vi "Send8Bytes.vi"(0 "data0":u8, 1 "data1":u8, 2 "data2":u8, 3 "data3":u8, 4 "data4":u8, 5 "data5":u8, 6 "data6":u8, 7 "data7":u8, 8 "类型":u32(ring)=4 items=["PCI5121"=1, "PCI9810"=2, "USBCAN1"=3, "USBCAN2"=4, "PCI9820"=5, "CAN232"=6, "PCI5110"=7, "CANLite(mini)"=8, "ISA9620"=9, "ISA5420"=10, "PC104CAN"=11, "CANET"=17, "DNP9810"=13, "USBCAN-E-U"=20, "USBCAN-2E-U"=21], 9 "板号/目标地址":u8, 10 "设备索引":u32(ring) items=["0", "1", "2", "3", "4", "5", "6", "7", "8", "9", "10", "11", "12", "13", "14", "15", ""], 12 "CAN路数":u32(ring) items=["0", "1"], 14 "ExternFlag":u8, 16 "ID":u32, 18 "DataLen":u8) -> (20 "发送状态":bool)   [LabVIEW 2013]
uses:
  BHN01/AutoBurn/Settings/ControlCAN.dll
panel:
  out "VCI_CAN_OBJ_T":T1 {"ID" format="%x"}
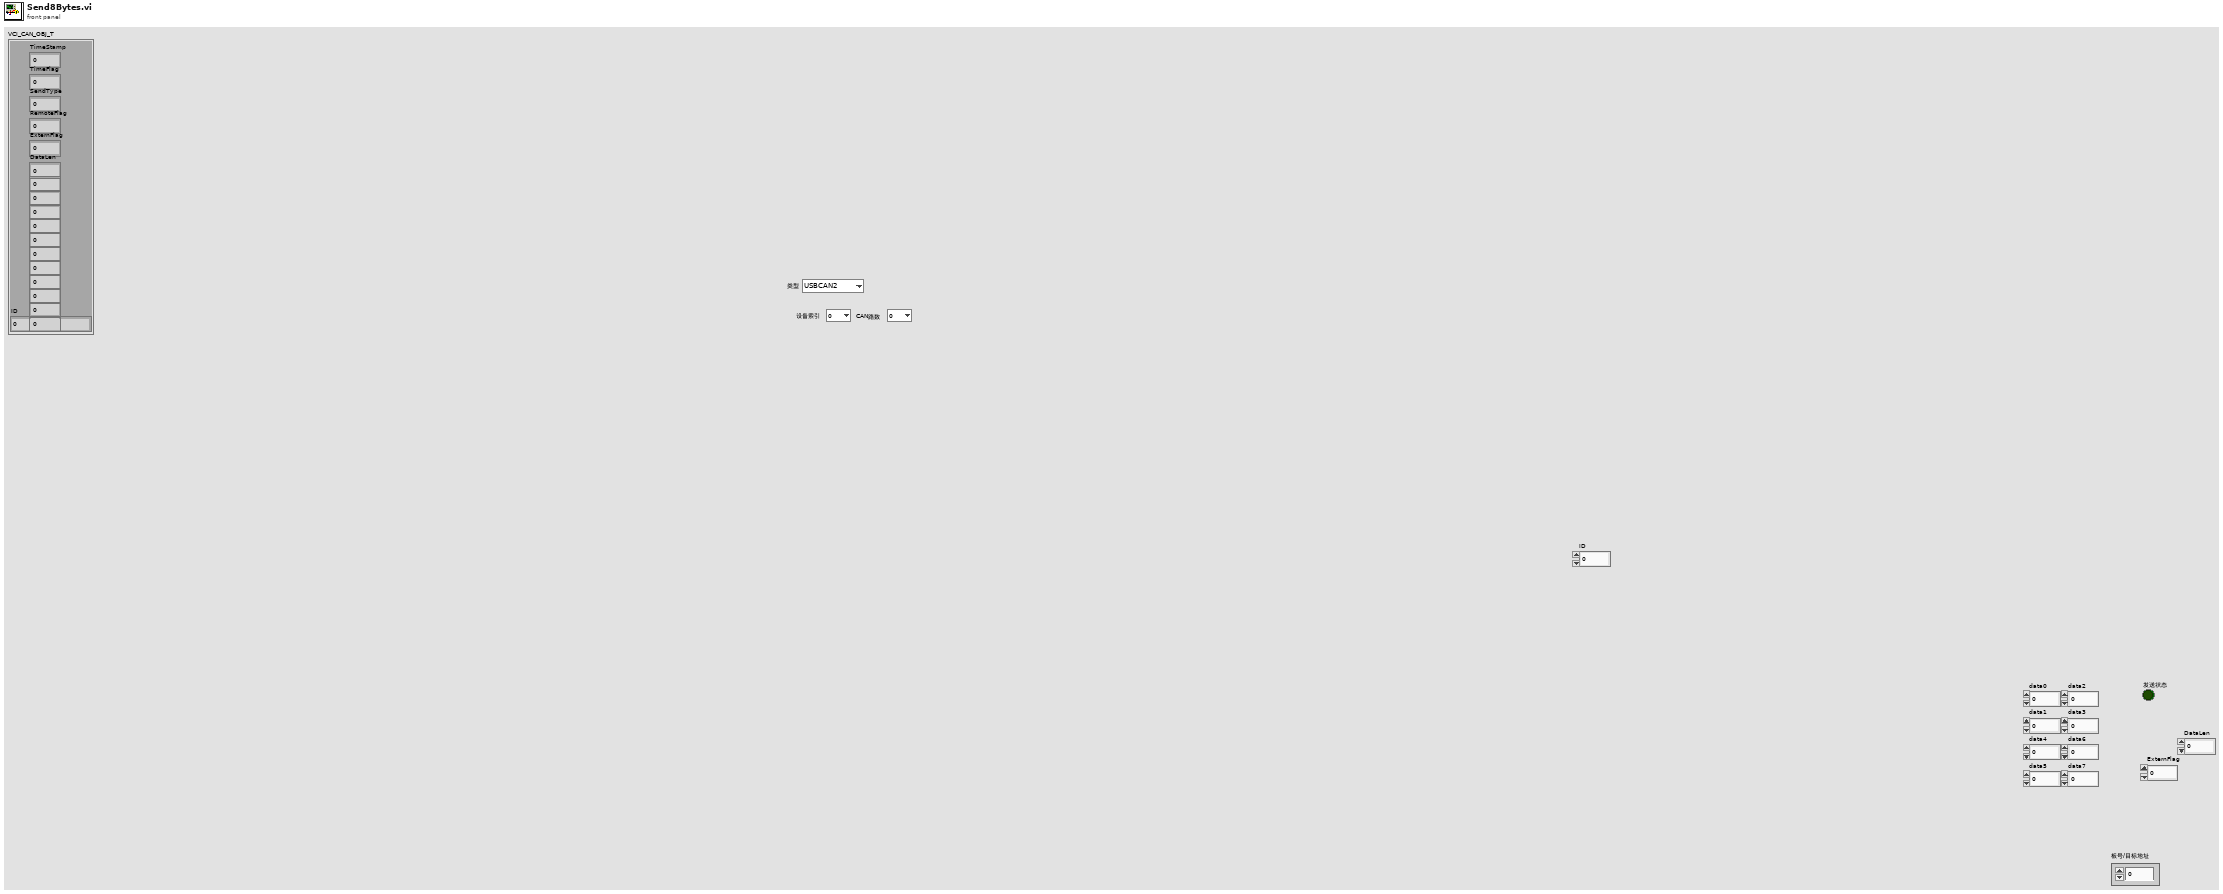
[diagram p1: front panel]
types:
  T1 = cluster{"ID":u32, "TimeStamp":u32, "TimeFlag":u8, "SendType":u8, "RemoteFlag":u8, "ExternFlag":u8, "DataLen":u8, u8, u8, u8, u8, u8, u8, u8, u8, u8, u8, u8}
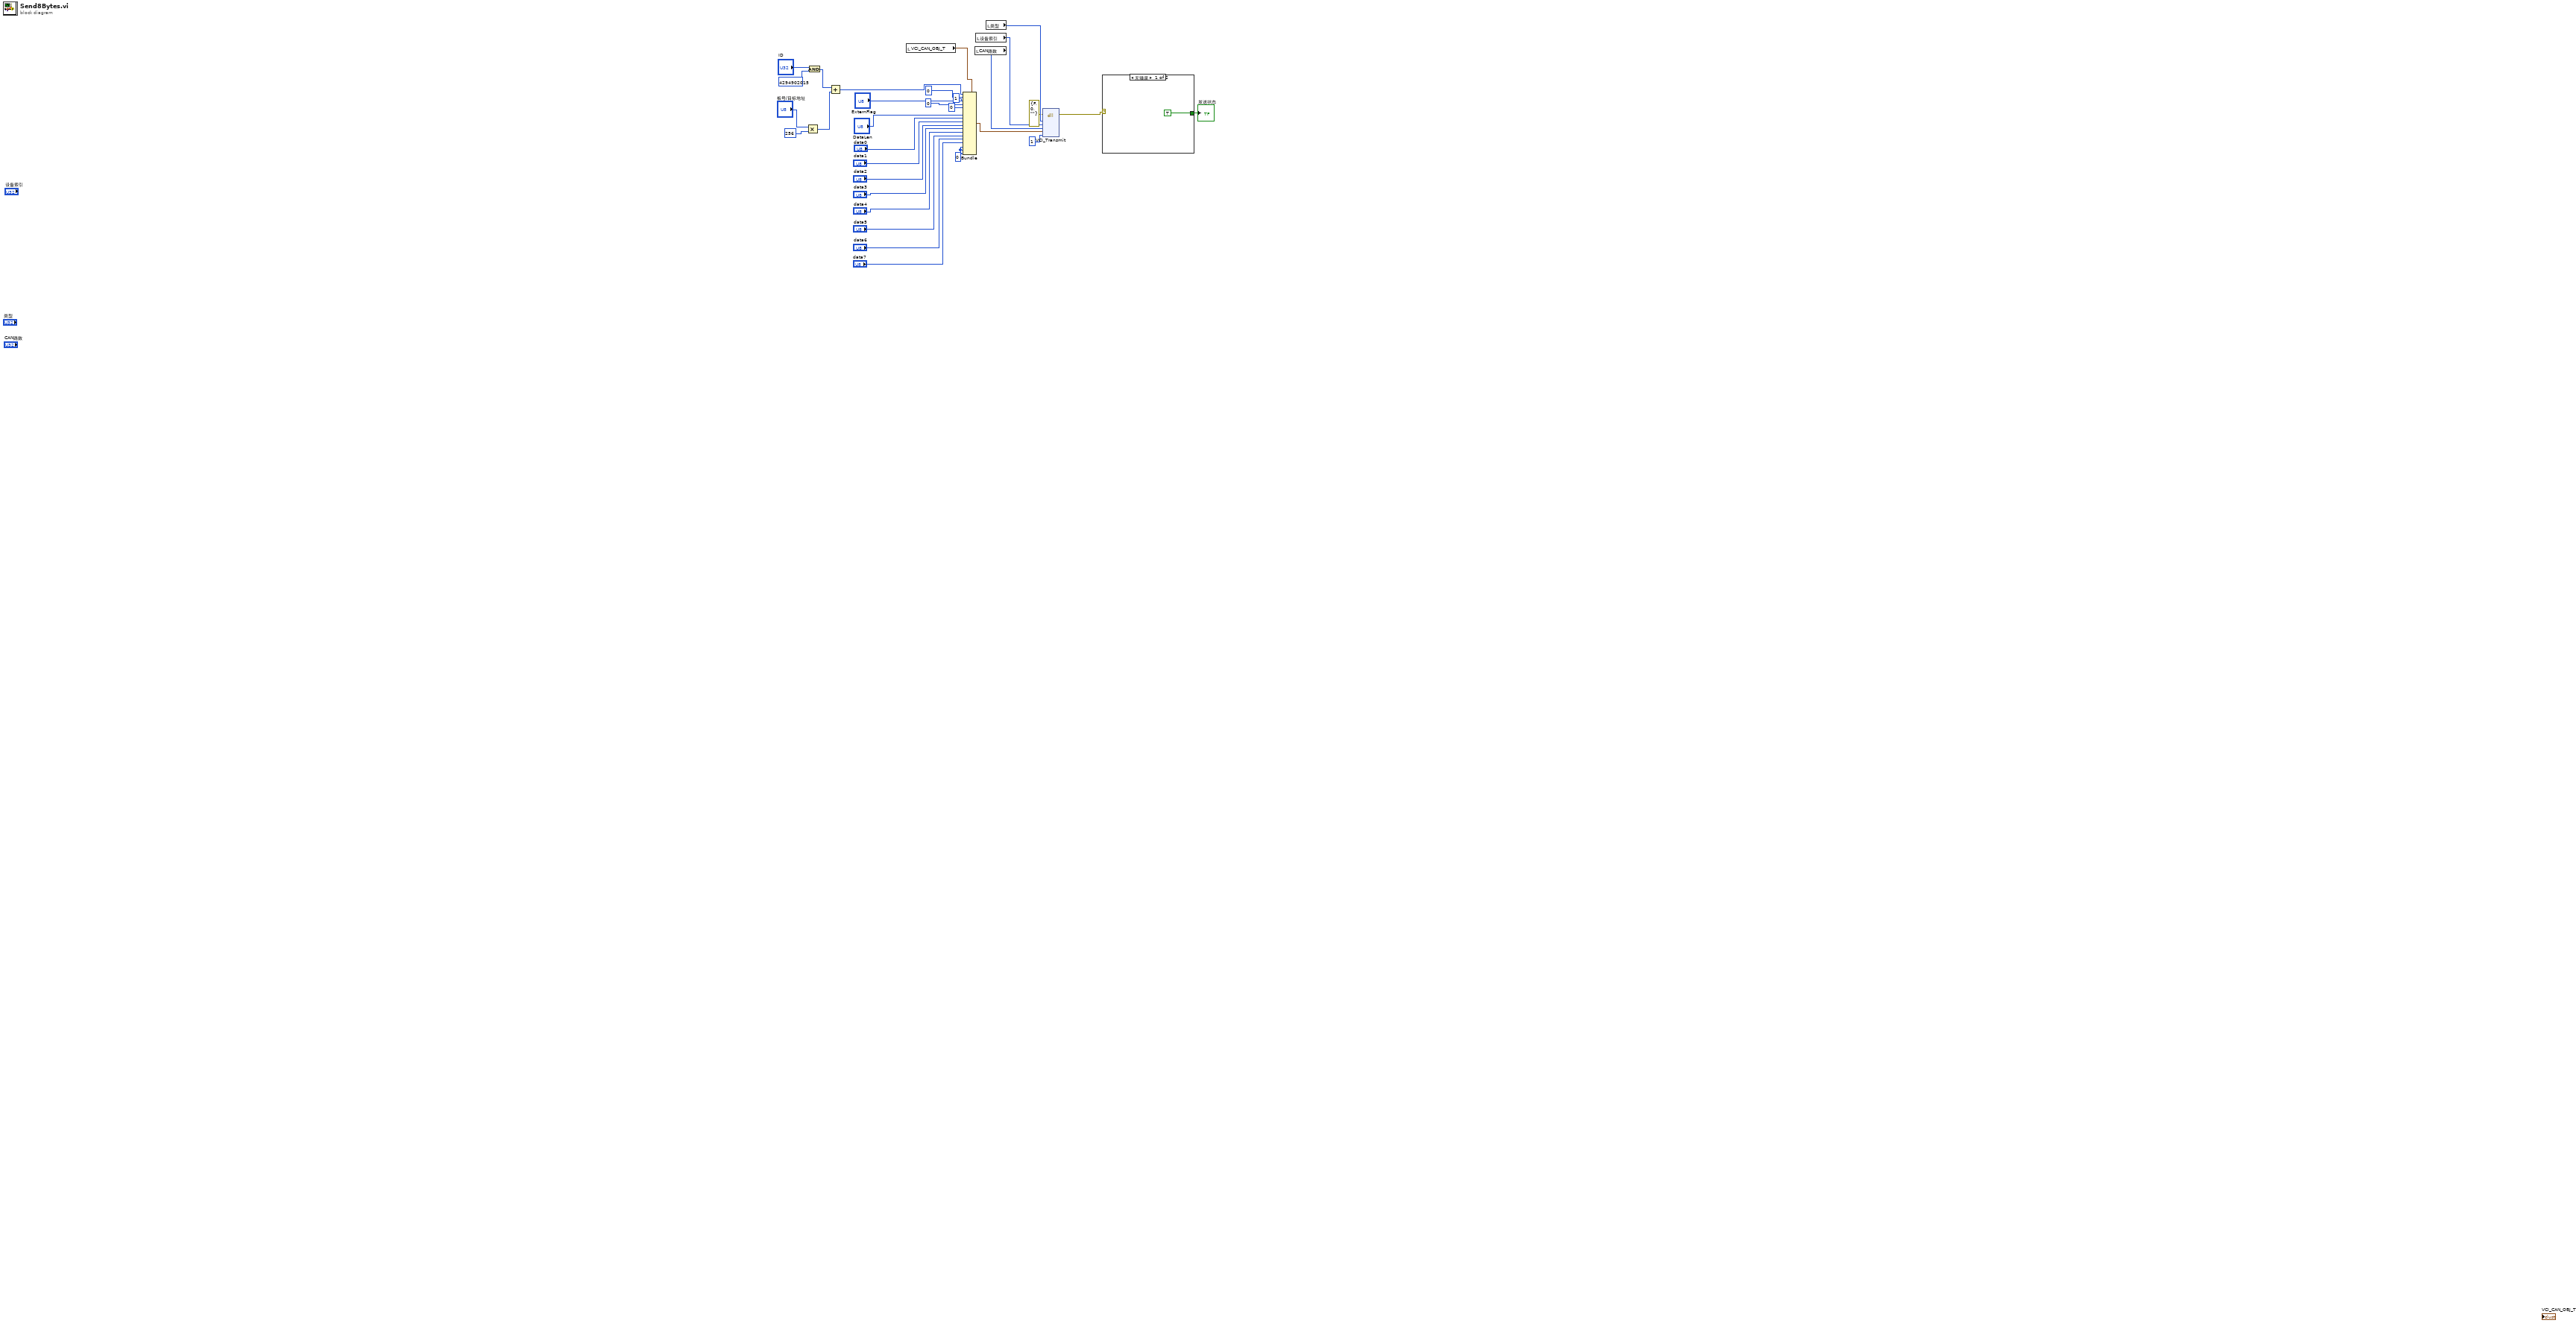
[diagram p0: block diagram]
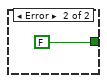
[diagram p2: hidden frame]
diagram:
  w22 = u8 0 ("元素")
  n1 = Multiply(x="板号/目标地址", y=u16 256) -> (x*y=w2:u16)
  n2 = And(x="ID", y=u32 4294902015) -> (x .and. y?=w6:u32)
  n3 = Add(x=w6, y=w2) -> (x+y=w5:u32)
  n4 = local read "VCI_CAN_OBJ_T"() -> (w26:T1)
  n5 = Bundle(cluster=w26, "ID"=w5, "TimeStamp"=u8 0 ("RemoteFlag"), "TimeFlag"=u8 1, "SendType"=u8 0 ("DataLen"), "RemoteFlag"=u8 0, "ExternFlag"="ExternFlag", "DataLen"="DataLen", "data0", "data1", "data2", "data3", "data4", "data5", "data6", "data7", w22, w22, w22) -> (w30:T1)
  n6 = local read "CAN路数"() -> (w27:u32)
  n7 = local read "设备索引"() -> (w28:u32)
  n8 = local read "类型"() -> (w29:u32)
  n9 = dll-call lib="F:/Bluewave New Energy/SVN_Work/AutoTest_TestStand/trunk/AutoTest_TestStand/Driver/ZlgCan/BHN01/AutoBurn/Settings/ControlCAN.dll" fn="VCI_Transmit"(error in=errorcluster {"status"=FALSE, "code"=0, "source"=""} ("错误输入（无错误）"), "DeviceType"=w29, "DeviceInd"=w28, "CANInd"=w27, "pSend"=w30, "Len"=u32 1) -> (error out=w17:errorcluster)  [unwired: 4 in, 5 out]
  n10 = case shown="无错误" w17 {
    tunnel: [TRUE FALSE] -> w16
    frame No Error {
    }
    frame Error {
    }
  }
  "发送状态" <- w16
